vi "ADS1115_Example.vi"() -> ()   [LabVIEW 2017]
uses:
  libMPSSE.lvlib
panel:
  out "(hi.lo) 2":u16 format="%.0b"
  out "x/y":dbl
  out "Data":u8[](array[numeric])
  out "mV out":dbl
  out "(hi.lo)":u16
  in  "options_i2c_write":T1
  out "Description":string
  out "Serial number":string
  in  "Config":T2={"ClockRate"=100000, "LatencyTimer"=1, "Disable 3 phase clocking"=FALSE, "Disable drive only 0"=FALSE} {"ClockRate" items=["I2C_CLOCK_STANDARD_MODE"=100000, "I2C_CLOCK_FAST_MODE"=400000, "I2C_CLOCK_FAST_MODE_PLUS"=1000000, "I2C_CLOCK_HIGH_SPEED_MODE"=3400000]}
  out "Waveform Chart":dbl[](graph)
  in  "stop":bool
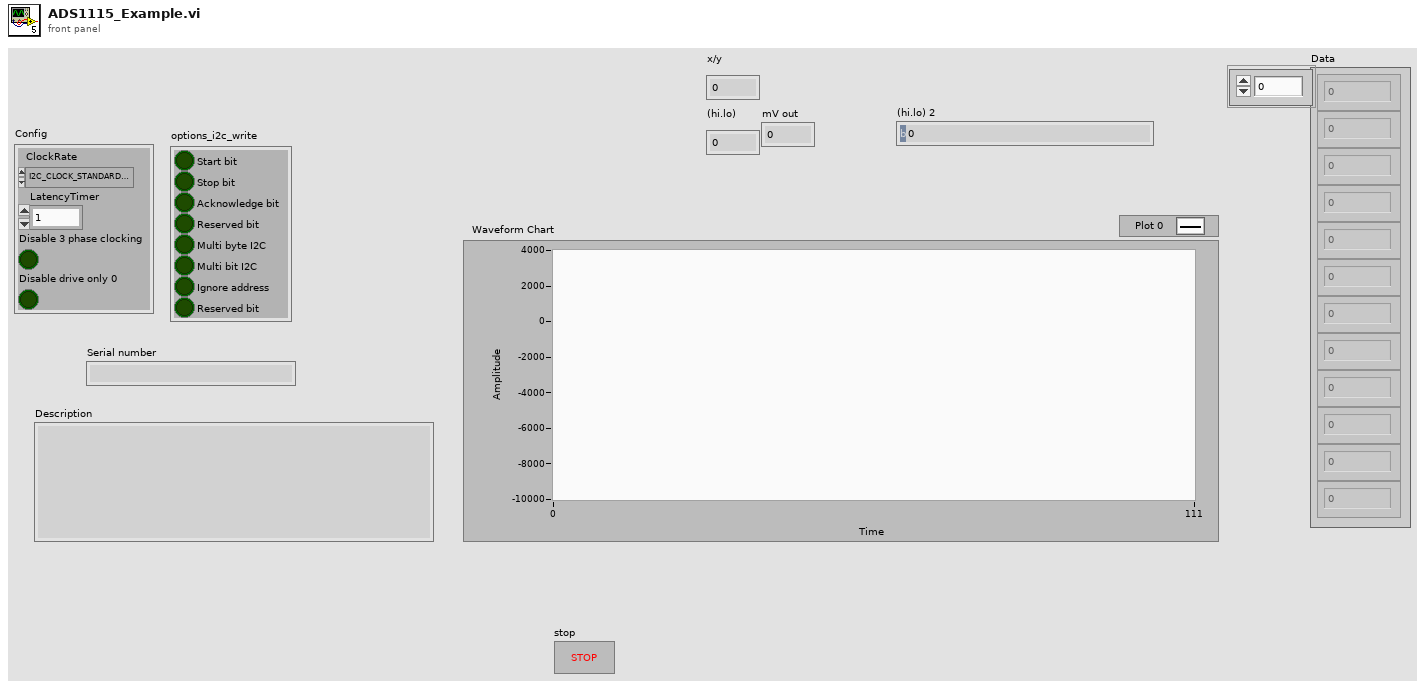
[diagram p1: front panel]
types:
  T1 = cluster{"Start bit":bool, "Stop bit":bool, "Acknowledge bit":bool, "Reserved bit":bool, "Multi byte I2C":bool, "Multi bit I2C":bool, "Ignore address":bool, "Reserved bit":bool}
  T2 = cluster{"ClockRate":u32, "LatencyTimer":u8, "Disable 3 phase clocking":bool, "Disable drive only 0":bool}
  T3 = cluster{"ADS1015-Channel Selector":enum8{"DIFF-AI0-AI1", "DIFF-AI0-AI3", "DIFF-AI1-AI3", "DIFF-AI2-AI3", "Single Ended - AI0", "Single Ended - AI1", "Single Ended - AI2", "Single Ended - AI3"}, "ADS1015 -Gain & Scale":enum8{"FS=+/-6.144 V", "FS=+/-4.096 V", "FS=+/-2.048 V", "FS=+/-1.024 V", "FS=+/-0.512 V", "FS=+/-0.256-A V", "FS=+/-0.256-B V", "FS=+/-0.256-C V"}, "ADS1015- Acquire Mode":enum16{"Continuous Conversion Mode", "Single Shot Mode"}, "ADS1015 Sample Rate":enum8{"128 SPS", "250 SPS", "490 SPS", "920 SPS", "1600 SPS", "2400 SPS", "3300 SPS", "3300 SPS A"}}
  T4 = enum8{"FS=+/-6.144 V", "FS=+/-4.096 V", "FS=+/-2.048 V", "FS=+/-1.024 V", "FS=+/-0.512 V", "FS=+/-0.256-A V", "FS=+/-0.256-B V", "FS=+/-0.256-C V"}
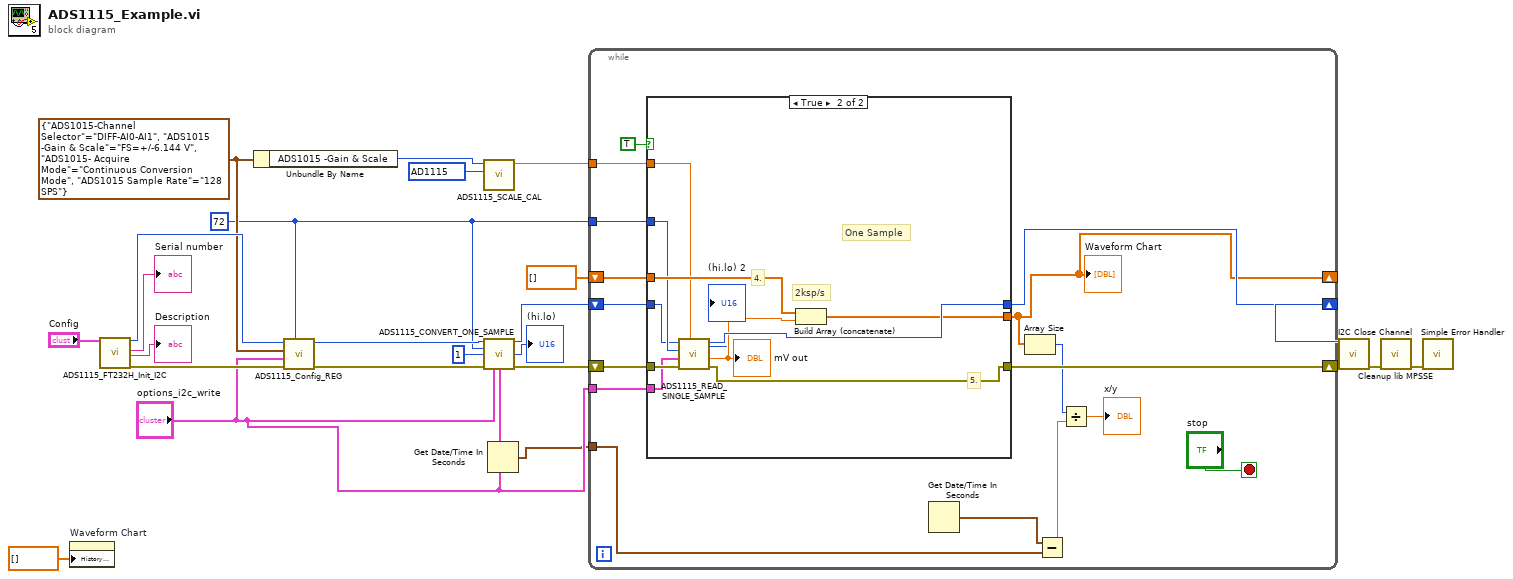
[diagram p0: block diagram]
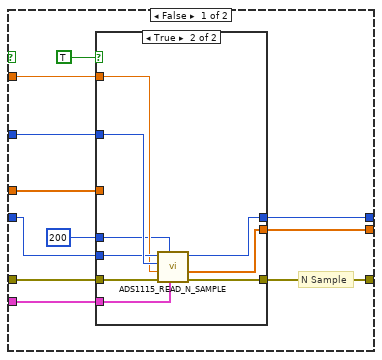
[diagram p2: hidden frame]
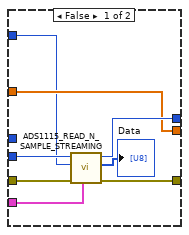
[diagram p3: hidden frame]
diagram:
  w7 = 65536 items=["ADS1015"=4096, "AD1115"=65536] ("IC Selector")
  w15 = u8 72 ("I2C Slave Address (0)")
  w18 = T3 {"ADS1015-Channel Selector"=enum."DIFF-AI0-AI1", "ADS1015 -Gain & Scale"=enum."FS=+/-6.144 V", "ADS1015- Acquire Mode"=enum."Continuous Conversion Mode", "ADS1015 Sample Rate"=enum."128 SPS"} ("ADS1015 Reg Config")
  n1 = property on="Waveform Chart" class="WFChart (strict)"("History Data"=dbl[] []) -> ()  [unwired: 2 in, 2 out]
  n2 = call "ADS1115_FT232H_Init_I2C.vi"("Config"="Config") -> ("handle out"=w20:u32, "Serial number"=→"Serial number":string, "Description"=→"Description":string, "error out"=w19:errorcluster)  [unwired: 15 in]
  n3 = Unbundle By Name(w18) -> ("ADS1015 -Gain & Scale"=w12:T4)
  n4 = call "ADS1115_Config_REG.vi"("I2C Slave Address (0) (ADS1115 Address)"=w15, "Error In"=w19, "options_i2c_write"="options_i2c_write", "ADS1015 Reg Config"=w18, "handle"=w20) -> ("Error Out"=w16:errorcluster, "handle out"=w17:u32)  [unwired: 5 in]
  n5 = call "ADS1115_SCALE_CAL.vi"("IC Selector"=w7, "ADS1015 -Gain & Scale"=w12) -> ("Scale Value (mV)"=w6:dbl)  [unwired: 9 in]
  n6 = call "ADS1115_CONVERT_ONE_SAMPLE.vi"("handle"=w17, "I2C Slave Address (0)"=w15, "Scale mV"=u16 1, "error in (no error)"=w16, "options_i2c_write"="options_i2c_write", "options_i2c_read"="options_i2c_write") -> ("handle out"=w13:u32, "(hi.lo)"=→"(hi.lo)":u16, "error out"=w14:errorcluster)  [unwired: 6 in, 1 out]
  n7 = Get Date/Time In Seconds() -> (seconds since 1Jan1904=w1:timestamp)
  n8 = while {
    shift-right: [w32] -> w10
    shift-left: w14 -> [w37]
    shift-right: [w30] -> _
    shift-left: dbl[] [] -> [w40]
    tunnel: w15 -> [w38]
    tunnel: w6 -> [w33]
    shift-right: [w34] -> w11
    shift-left: w13 -> [w35]
    tunnel: "options_i2c_write" -> [w36]
    tunnel: w1 -> [w28]
    stop <- "stop" stop-if-true
    n9 = case shown="True" TRUE {
      tunnel: w40 -> [w42 w79]
      tunnel: w38 -> [w46 w78]
      tunnel: w37 -> [w48 w77]
      tunnel: w36 -> [w47 w76]
      tunnel: w35 -> [w45 w75]
      tunnel: [w50 w74] -> w34
      tunnel: w33 -> [w44 w72]
      tunnel: [w49 w71] -> w32
      tunnel: [w51 w70] -> w30
      frame False {
        # "N Sample"
        n10 = case shown="True" TRUE {
          tunnel: [w54 w68] -> w51
          tunnel: [w56 w67] -> w50
          tunnel: [w59 w66] -> w49
          tunnel: w48 -> [w58 w65]
          tunnel: w47 -> [w53 w64]
          tunnel: w46 -> [w52 w63]
          tunnel: w45 -> [w57 w62]
          tunnel: w44 -> [_ w61]
          tunnel: u32 200 ("N_Samples") -> [_ w60]
          tunnel: w42 -> [w54 _]
          frame False {
            n11 = call "ADS1115_READ_N_SAMPLE_STREAMING.vi"("options_i2c_read"=w53, "error in (no error)"=w58, "I2C Slave Address (0)"=w52, "handle"=w57) -> ("error out"=w59:errorcluster, "Data read"=→"Data":u8[], "handle out"=w56:u32)  [unwired: 5 in]
          }
          frame True {
            n12 = call "ADS1115_READ_N_SAMPLE.vi"("options_i2c_read"=w64, "N_Samples"=w60, "error in (no error)"=w65, "Scale Value (mV)"=w61, "I2C Slave Address (0)"=w63, "handle"=w62) -> ("error out"=w66:errorcluster, "mV"=w68:dbl[], "handle out"=w67:u32)  [unwired: 2 in, 1 out]
          }
        }
      }
      frame True {
        # "One Sample"
        # "2ksp/s"
        # "5."
        # "4."
        n13 = call "ADS1115_READ_SINGLE_SAMPLE.vi"("Scale Value (mV)"=w72, "error in (no error)"=w77, "options_i2c_read"=w76, "I2C Slave Address (0)"=w78, "handle"=w75) -> ("error out"=w71:errorcluster, "mV out"=w73:dbl, "handle out"=w74:u32, "(hi.lo)"=→"(hi.lo) 2":u16)  [unwired: 1 in, 2 out]
        "mV out" <- w73
        n14 = Build Array (concatenate)(w79, w73) -> (w70:dbl[])
      }
    }
    "Waveform Chart" <- w30
    n15 = Get Date/Time In Seconds() -> (seconds since 1Jan1904=w29:timestamp)
    n16 = Array Size(array=w30) -> (size(s)=w26:i32)
    n17 = Subtract(x=w29, y=w28) -> (x-y=w27:dbl)
    n18 = Divide(x=w26, y=w27) -> (x/y=→"x/y":dbl)
  }
  n19 = call "I2C Close Channel.vi"("handle"=w11, "error in (no error)"=w10) -> ("error out"=w9:errorcluster)  [unwired: 13 in]
  n20 = call "Cleanup lib MPSSE.vi"("error in (no error)"=w9) -> ("error out"=w8:errorcluster)  [unwired: 14 in]
  n21 = call <vilib>:"Simple Error Handler.vi"("error in (no error)"=w8) -> ()  [unwired: 4 in, 5 out]
